vi "CanTran.vi"(6 "error in (no error)":errorcluster, 7 "CanIndex":u32, 8 "Reserved":u32, 9 "DevIndex":u32, 10 "DevType":u32(ring) items=["null", "VCI_PCI5121", "VCI_PCI9810", "VCI_USBCAN1", "VCI_USBCAN2", "VCI_PCI9820", "VCI_CAN232", "VCI_PCI5110", "VCI_CANLITE", "VCI_ISA9620", "VCI_ISA5420", "VCI_PC104CAN", "VCI_CANETE", "VCI_DNP9810", "VCI_PCI9840", "PC104-CAN2 ", "VCI_PCI9820I "]) -> (1 "CANIndex":u32, 2 "DevIndex 2":u32, 3 "DevType 2":u32, 4 "success?":T2, 5 "error out":errorcluster)   [LabVIEW 2014]
uses:
  ControlCAN.dll
panel:
  in  "pInit_Config":T1
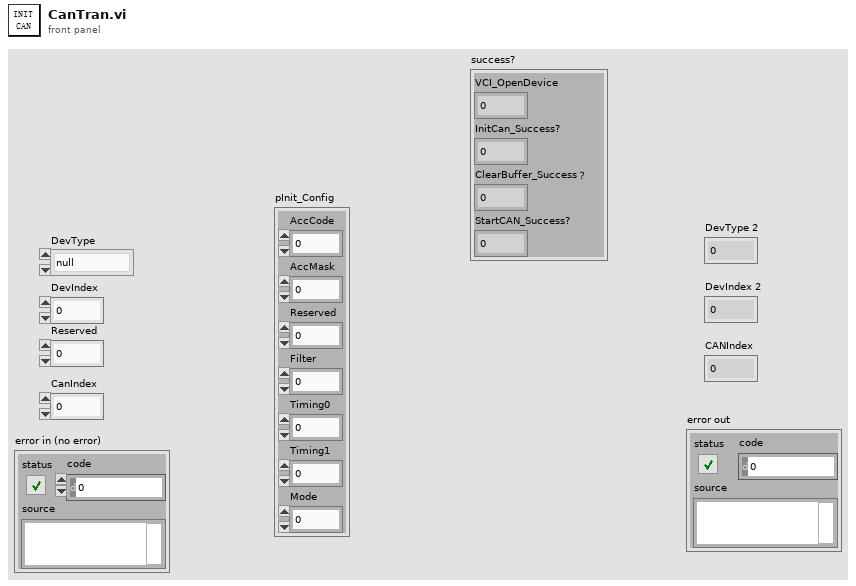
[diagram p1: front panel]
types:
  T1 = cluster{"AccCode":u32, "AccMask":u32, "Reserved":u32, "Filter":u8, "Timing0":u8, "Timing1":u8, "Mode":u8}
  T2 = cluster{"VCI_OpenDevice":u32, "InitCan_Success?":u32, "ClearBuffer_Success？":u32, "StartCAN_Success?":u32}
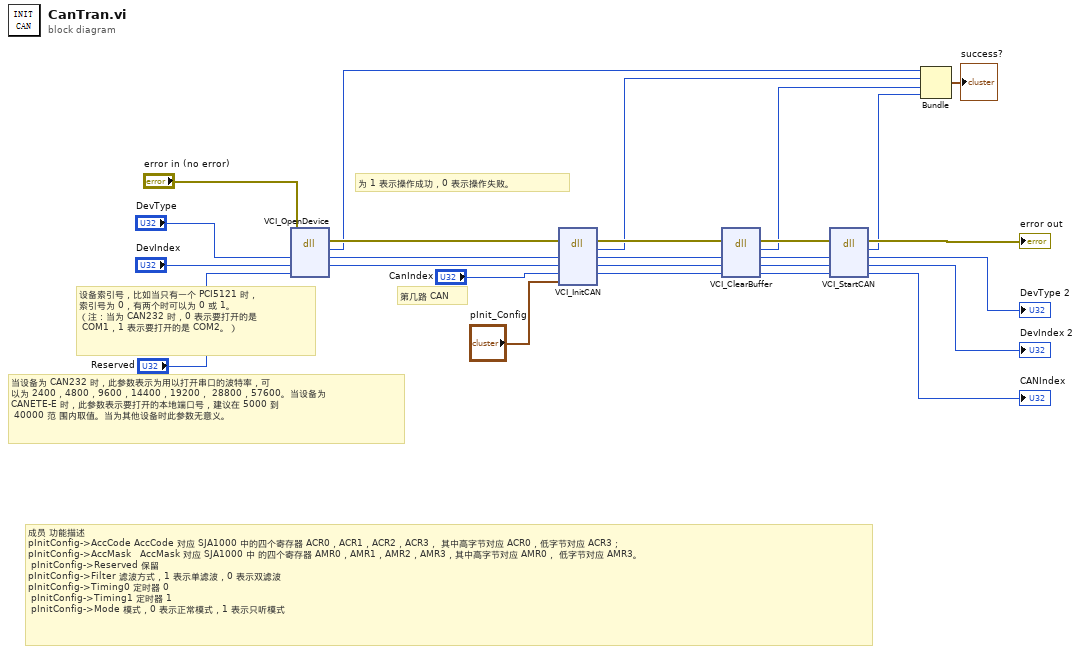
[diagram p0: block diagram]
diagram:
  # "成员 功能描述 \npInitConfig->AccCode AccCode 对应 SJA1000 中的四个寄存器 ACR0，ACR1，ACR2，ACR3， 其中高字节对应 ACR0，低字节对应 ACR3；  \npInitConfig->AccMask   AccMask 对应 SJA1000 中 的四个寄存器 AMR0，AMR1，AMR2，AMR3，其中高字节对应 AMR0， 低字节对应 AMR3。\n pInitConfig->Reserved 保留 \npInitConfig->Filter 滤波方式，1 表示单滤波，0 表示双滤波 \npInitConfig->Timing0 定时器 0\n pInitConfig->Timing1 定时器 1\n pInitConfig->Mode 模式，0 表示正常模式，1 表示只听模式"
  # "第几路 CAN"
  # "为 1 表示操作成功，0 表示操作失败。"
  # "设备索引号，比如当只有一个 PCI5121 时，\n索引号为 0，有两个时可以为 0 或 1。 \n（注：当为 CAN232 时，0 表示要打开的是\n COM1，1 表示要打开的是 COM2。）"
  # "当设备为 CAN232 时，此参数表示为用以打开串口的波特率，可\n以为 2400，4800，9600，14400，19200， 28800，57600。当设备为 \nCANETE-E 时，此参数表示要打开的本地端口号，建议在 5000 到\n 40000 范 围内取值。当为其他设备时此参数无意义。"
  n1 = dll-call lib="PTH22abs D\tDocuments\tCan总线canControlCAN.dll" fn="VCI_OpenDevice"(error in="error in (no error)", "DevType"="DevType", "DevIndex"="DevIndex", "Reserved"="Reserved") -> (error out=w21:errorcluster, "VCI_OpenDevice"=w6:u32, "DevType"=w24:u32, "DevIndex"=w23:u32)  [unwired: 3 in, 1 out]
  n2 = dll-call lib="PTH22abs D\tDocuments\tCan总线canControlCAN.dll" fn="VCI_InitCAN"(error in=w21, "DevType"=w24, "DevIndex"=w23, "CanIndex"="CanIndex", "pInit_Config"="pInit_Config") -> (error out=w13:errorcluster, "InitCan_Success?"=w5:u32, "DevType"=w14:u32, "DevIndex"=w15:u32, "CanIndex"=w16:u32)  [unwired: 3 in, 1 out]
  n3 = dll-call lib="PTH22abs D\tDocuments\tCan总线canControlCAN.dll" fn="VCI_ClearBuffer"(error in=w13, "DevType"=w14, "DevIndex"=w15, "CANIndex"=w16) -> (error out=w12:errorcluster, "ClearBuffer_Success？"=w4:u32, "DevType"=w19:u32, "DevIndex"=w18:u32, "CANIndex"=w17:u32)  [unwired: 2 in, 1 out]
  n4 = dll-call lib="PTH22abs D\tDocuments\tCan总线canControlCAN.dll" fn="VCI_StartCAN"(error in=w12, "DevType"=w19, "DevIndex"=w18, "CANIndex"=w17) -> (error out=→"error out":errorcluster, "StartCAN_Success?"=w3:u32, "DevType"=→"DevType 2":u32, "DevIndex"=→"DevIndex 2":u32, "CANIndex"=→"CANIndex":u32)  [unwired: 2 in, 1 out]
  n5 = Bundle("VCI_OpenDevice"=w6, "InitCan_Success?"=w5, "ClearBuffer_Success？"=w4, "StartCAN_Success?"=w3) -> (→"success?":T2)  [unwired: 1 in]
